vi "Get Data String.vi"(8 "error in":errorcluster, 11 "CAN Message in":refnum<class "CAN Message.lvclass">) -> (0 "error out":errorcluster, 2 "Data String":string, 3 "CAN Message out":refnum<class "CAN Message.lvclass">)   [LabVIEW 2025, in "CAN Message.lvclass"]
uses:
  CAN Message.lvclass
  CAN Message.lvclass/CAN Message.ctl
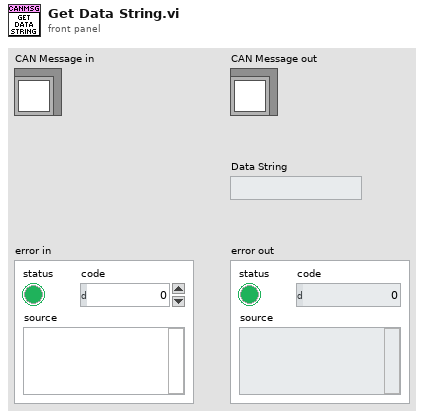
[diagram p1: front panel]
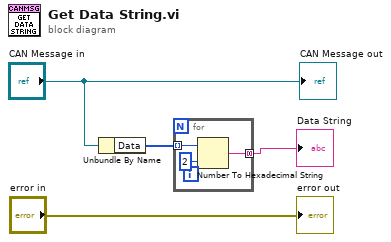
[diagram p0: block diagram]
diagram:
  n1 = Unbundle By Name("CAN Message in") -> ("Data"=w2:u8[])
  n2 = for {
    tunnel: w2 -> [w7] mode=indexing
    tunnel: [w5] -> w1 mode=concatenating
    n3 = Number To Hexadecimal String(1:i16 2 ("width (-)"), 2:w7) -> (0:w5:string)
  }
  "Data String" <- w1
  "CAN Message out" <- "CAN Message in"
  "error out" <- "error in"
